vi "CurrentInput_flt.vi"(6 "maxforcey":dbl, 8 "Mode":u16(ring) items=["Log w/ Exp Z", "Log w/ Lin Z"], 9 "Maximum (pA)":dbl=9000.0, 10 "Current (pA)":dbl format="%.1f", 11 "Setpoint (A)":dbl=100.0) -> (2 "Setpoint (pA)":dbl, 3 "Filtered Current (pA)":dbl format="%.1f", 7 "Safetip?":bool)   [LabVIEW 2019]
uses:
  <vilib>/Analysis/3filter.llb/Filter Passband Type.ctl
  <userlib>/HapticSTM/HapticSTM.lvlib
  <vilib>/ptbypt/NI_PtbyPt.lvlib
  <vilib>/Analysis/NI_AALBase.lvlib
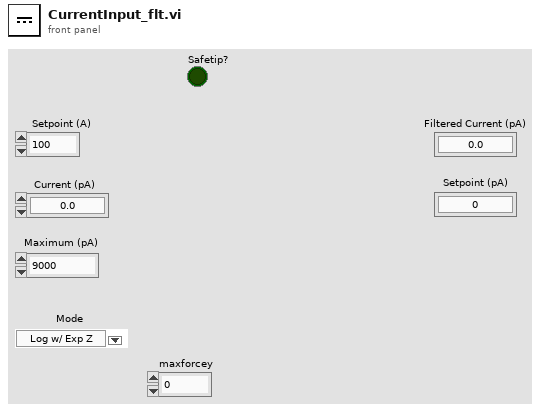
[diagram p1: front panel]
types:
  T1 = typedef "NI_AALBase.lvlib/Filter Passband Type.ctl" = enum32{"Lowpass", "Highpass", "Bandpass", "Bandstop"}
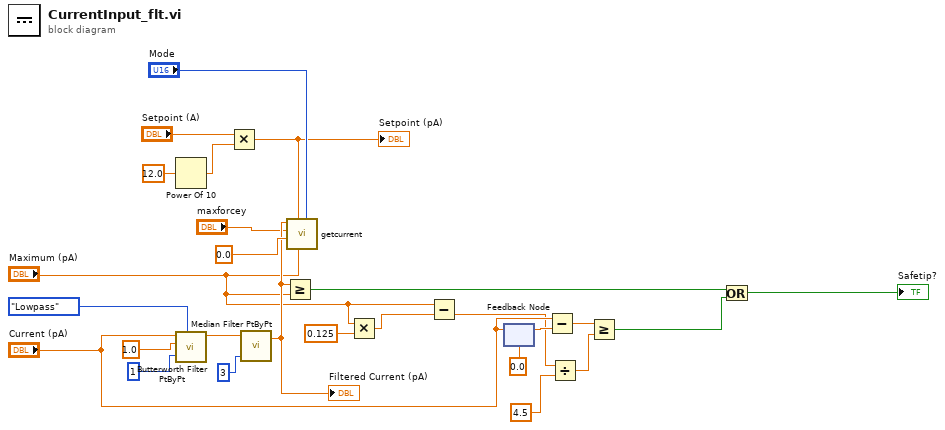
[diagram p0: block diagram]
diagram:
  n1 = Power Of 10(x=12.0) -> (10^x=w25:dbl)
  n2 = call <vilib>:"Butterworth Filter PtByPt.vi"("order"=1, "filter type"=Filter_Passband_Type."Lowpass", "sampling freq: fs"=1.0, "x"="Current (pA)") -> ("Filtered x"=w20:dbl)  [unwired: 5 in, 1 out]
  n3 = Multiply(x="Setpoint (A)", y=w25) -> (x*y=w16:dbl)
  "Setpoint (pA)" <- w16
  n4 = call <vilib>:"Median Filter PtByPt.vi"("rank"=3, "x"=w20) -> ("Filtered x"=w15:dbl)  [unwired: 2 in, 1 out]
  "Filtered Current (pA)" <- w15
  n5 = Greater Or Equal?(x=w15, y="Maximum (pA)") -> (x >= y?=w17:bool)
  n6 = call <userlib>:"getcurrent.vi"("forcemode"="Mode", "maxcurrentin"="Maximum (pA)", "setpoint"=w16, "minforcey"=0.0, "maxforcey"="maxforcey", "currentin"=w15) -> ()  [unwired: 6 in]
  n7 = Multiply(x="Maximum (pA)", y=0.125) -> (x*y=w2:dbl)
  n8 = Subtract(x="Maximum (pA)", y=w2) -> (x-y=w5:dbl)
  n9 = feedback-in #1("Current (pA)") -> ()
  n10 = feedback #1(0.0 ("Current (pA)")) -> (w12:dbl)
  n11 = Subtract(x="Current (pA)", y=w12) -> (x-y=w9:dbl)
  n12 = Divide(x=w5, y=4.5) -> (x/y=w7:dbl)
  n13 = Greater Or Equal?(x=w9, y=w7) -> (x >= y?=w8:bool)
  n14 = Or(x=w17, y=w8) -> (x .or. y?=→"Safetip?":bool)
